vi "CurrentTest.vi"(0 "datain":string[](array[string])=["备注", "负载通道", "负载地址", "延时时间", "output max", "output min", "量测类型", "待测物板号"], 5 "HW CH Number":i32, 7 "Setup":string) -> (4 "REPORT INDECATE":string[][](array[string])=[["微安测试", "", "", "", ""], ["微安量测", "4", "0.000", "0.1", "NG"], ["微安量测", "4", "0.000", "0.1", "NG"], ["微安量测", "4", "0.000", "0.1", "NG"], ["微安量测", "4", "0.000", "0.1", "NG"]], 6 "ROW HEAD":string[](array[string]), 8 "PF":string[](array[string]), 10 "testData":string[](array[string]), 14 "数组":bool[](array[boolean]), 15 "Array":string[](array[string]))   [LabVIEW 2018]
panel:
  out "测试板数":i32
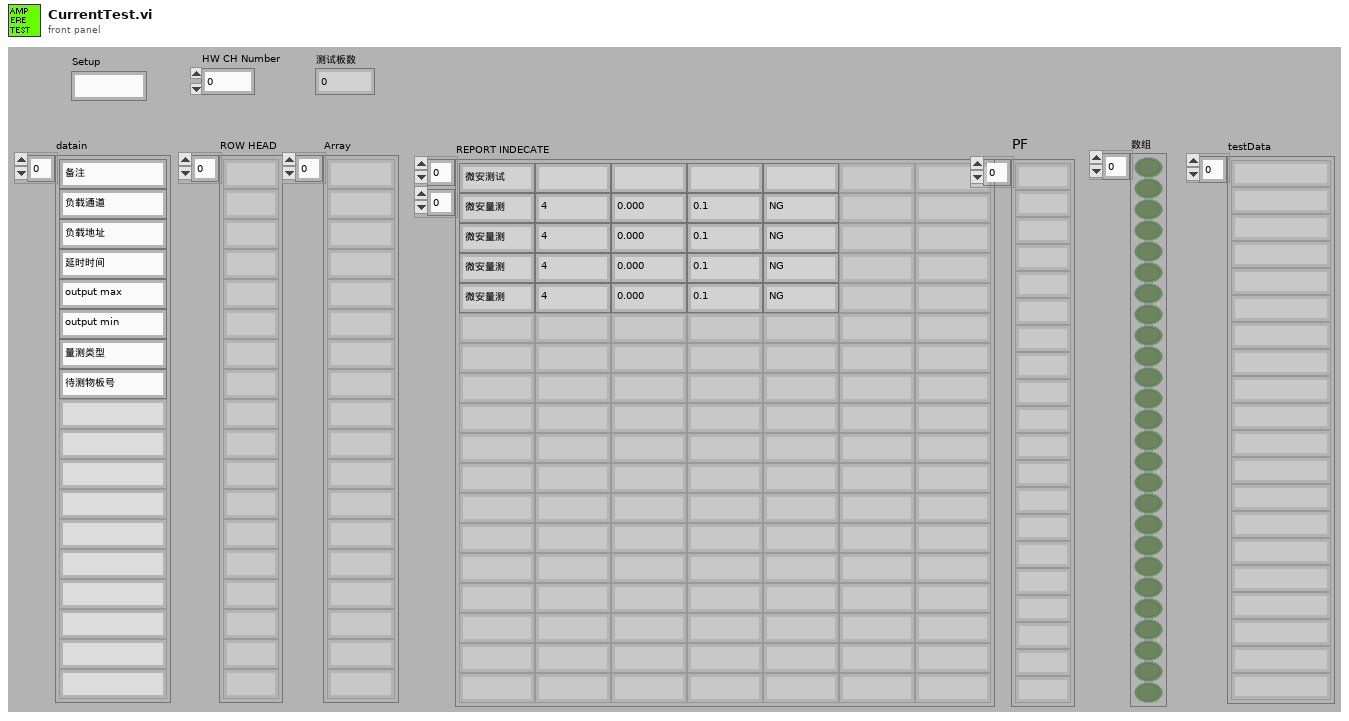
[diagram p1: front panel]
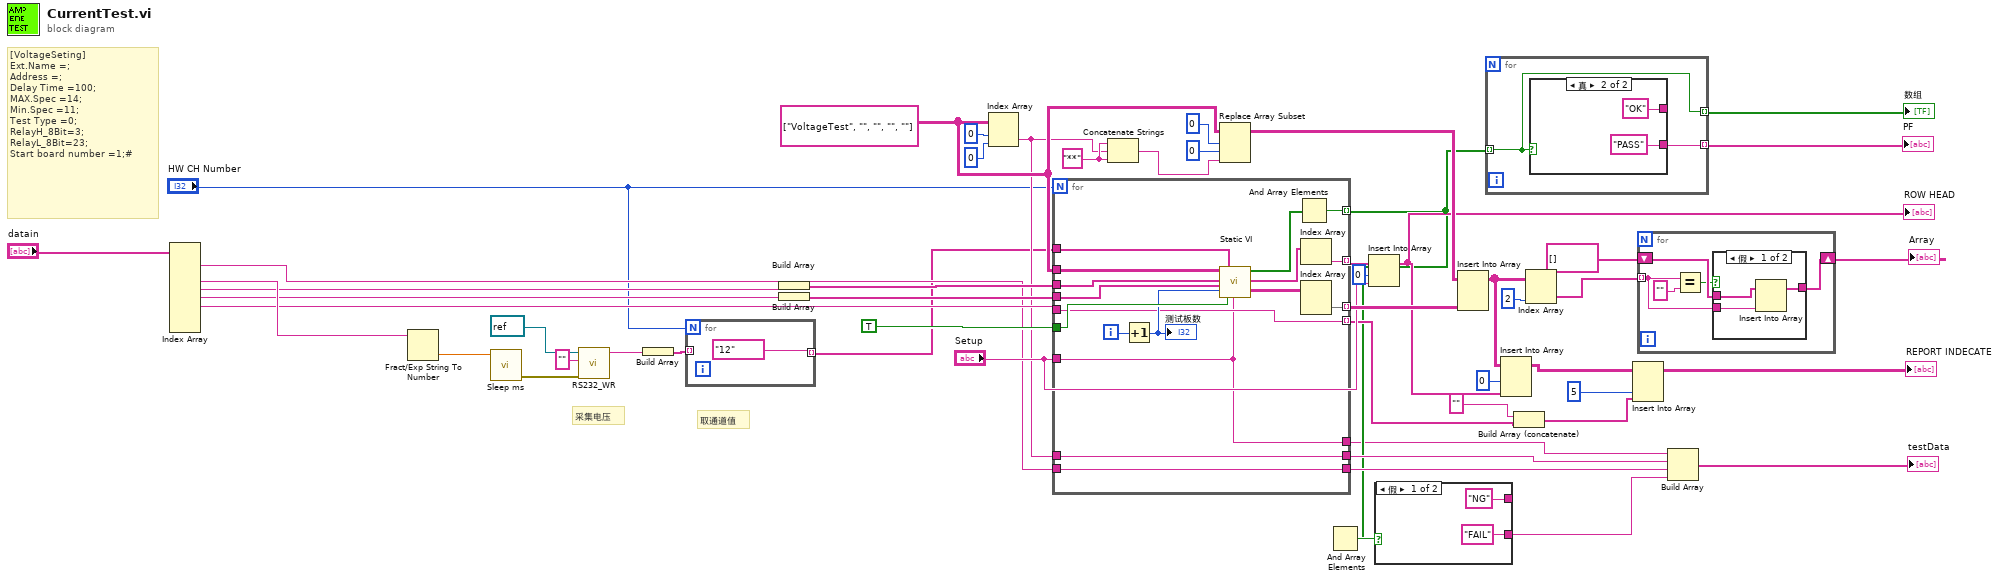
[diagram p0: block diagram]
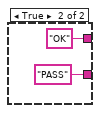
[diagram p2: hidden frame]
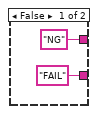
[diagram p3: hidden frame]
diagram:
  w37 = string[][] [["VoltageTest", "", "", "", ""]]
  w43 = "**" ("字符串")
  # "取通道值"
  # "采集电压"
  # "[VoltageSeting]\nExt.Name =;\nAddress =;\nDelay Time =100;\nMAX.Spec =14;\nMin.Spec =11;\nTest Type =0;\nRelayH_8Bit=3;\nRelayL_8Bit=23;\nStart board number =1;#"
  n1 = Index Array(array="datain") -> (element #1=w17:string, element #3=w46:string, element #4=w39:string, element #5=w38:string, element #6=w25:string)  [unwired: 9 in, 4 out]
  n2 = Fract/Exp String To Number(string=w46) -> (number=w1:dbl)  [unwired: 3 in, 1 out]
  n3 = call "Sleep ms.vi"("等待时间（毫秒）"=w1) -> ("error out"=w6:errorcluster)  [unwired: 10 in]
  n4 = call "RS232_WR.vi"("error in (no error)"=w6, "CMD"="", "VISA资源名称"=refnum<visa-resource-name> refnum) -> ("读取缓冲区"=w5:string)  [unwired: 6 in, 2 out]
  n5 = Build Array(w5) -> (w4:string[])
  n6 = for {
    N: "HW CH Number" -> [_]
    tunnel: w4 -> [_] mode=indexing
    tunnel: ["12" ("F-格式字符串")] -> w2 mode=indexing
  }
  n7 = Build Array(w39) -> (w36:string[])
  n8 = Build Array(w38) -> (w35:string[])
  n9 = Index Array(array=w37, index (row)=0 ("索引 (行)"), index (col)=0 ("禁用的索引 (列)")) -> (element=w18:string)
  n10 = for {
    N: "HW CH Number" -> [_]
    tunnel: w2 -> [w70]
    tunnel: w36 -> [w68]
    tunnel: w35 -> [w67]
    tunnel: "Setup" -> [w54]
    tunnel: TRUE -> [w65]
    tunnel: [w63] -> w13 mode=indexing
    tunnel: [w60] -> w31 mode=indexing
    tunnel: w37 -> [w69]
    tunnel: [w58] -> w32 mode=indexing
    tunnel: w25 -> [w57]
    tunnel: [w57] -> w21 mode=indexing
    tunnel: w18 -> [w56]
    tunnel: [w56] -> w16
    tunnel: w17 -> [w55]
    tunnel: [w55] -> w15
    tunnel: [w54] -> w10
    i -> [w62]
    n11 = Increment(x=w62) -> (x+1=w64:i32)
    "测试板数" <- w64
    n12 = call "Static VI.vi"("添加的数组"=w69, "Max"=w68, "Min"=w67, "板数"=w64, "INPUTSTRING"=w70, "是否为字符串对比"=w65, "SQ"=w54) -> ("P/F"=w66:bool[], "SQ out"=w61:string[], "arrauy out"=w59:string[][])  [unwired: 9 in, 1 out]
    n13 = And Array Elements(Boolean array=w66) -> (logical AND=w63:bool)
    n14 = Index Array(array=w61) -> (element=w60:string)  [unwired: 1 in]
    n15 = Index Array(array=w59) -> (element=w58:string[])  [unwired: 2 in]
  }
  n16 = Concatenate Strings(w43, w18, w43) -> (w40:string)
  n17 = Replace Array Subset(array=w37, new element=w40, index (row)=0 ("索引 (行)"), index (col)=0 ("禁用的索引 (列)")) -> (w33:string[][])
  n18 = And Array Elements(Boolean array=w13) -> (logical AND=w14:bool)
  n19 = Insert Into Array(array=w31, index=0 ("索引"), new element="Setup") -> (w27:string[])
  "ROW HEAD" <- w27
  n20 = case shown="假" w14 {
    tunnel: ["NG" "OK"] -> _
    tunnel: ["FAIL" "PASS"] -> w12
    frame False {
    }
    frame True {
    }
  }
  n21 = Insert Into Array ("数组插入")(array=w33, new element=w32) -> (w28:string[][])  [unwired: 2 in]
  n22 = for {
    tunnel: w13 -> [w75] mode=indexing
    tunnel: [w76] -> w48 mode=indexing
    tunnel: [w75] -> w9 mode=indexing
    n23 = case shown="真" w75 {
      tunnel: ["NG" "OK"] -> _
      tunnel: ["FAIL" "PASS"] -> w76
      frame False {
      }
      frame True {
      }
    }
  }
  "PF" <- w48
  "数组" <- w9
  n24 = Insert Into Array(array=w28, index (col)=0 ("禁用的索引 (列)"), new element=w27) -> (w23:string[][])  [unwired: 1 in]
  n25 = Build Array (concatenate)("" ("字符串"), w21) -> (w19:string[])
  n26 = Index Array(array=w28, index (col)=2 ("禁用的索引 (列)")) -> (element=w50:string[])  [unwired: 1 in]
  n27 = Insert Into Array(array=w23, index (col)=5 ("禁用的索引 (列)"), new element=w19) -> (→"REPORT INDECATE":string[][])  [unwired: 1 in]
  n28 = for {
    tunnel: w50 -> [w81] mode=indexing
    shift-right: [w82] -> w49
    shift-left: string[] [] ("Array") -> [w85]
    n29 = Equal?(x=w81, y="") -> (x = y?=w83:bool)
    n30 = case shown="假" w83 {
      tunnel: w85 -> [w88 w89]
      tunnel: [w87 w89] -> w82
      tunnel: w81 -> [w86 _]
      frame False {
        n31 = Insert Into Array(array=w88, new element=w86) -> (w87:string[])  [unwired: 1 in]
      }
      frame True {
      }
    }
  }
  "Array" <- w49
  n32 = Build Array(w10, w16, w15, w12) -> (→"testData":string[])
